vi "SavePosition_KCubeDCServo.vi"(4 "start/stop write":bool, 5 "init file":bool, 7 "Device":refnum<k24>, 8 "state in":T1(ring), 9 "filename save":string="D:\\Victor Sun\\optical trap control\\output_test\\testposition", 10 "folder path save":path, 11 "Byte Stream File in":refnum<file>) -> (0 "state out":T1(ring), 2 "current state":string, 3 "Byte Stream File out":refnum<file>)   [LabVIEW 2019]
doc: "saves datetime, position value, and isdevicebusy for dcservo motor"
uses:
  D:/Victor Sun/optical trap control/Kinesis/ThorLabs.MotionControl.KCube.DCServoCLI.dll
  Kinesis/ThorLabs.MotionControl.KCube.DCServoCLI.dll
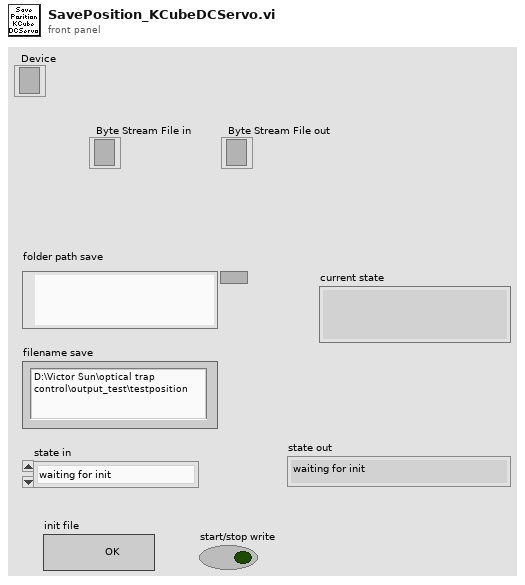
[diagram p1: front panel]
types:
  T1 = enum16{"waiting for init", "init", "waiting for write", "write", "stop", ""}
  T2 = enum16{"open", "replace", "create", "open or create", "replace or create", "replace or create with confirmation"}
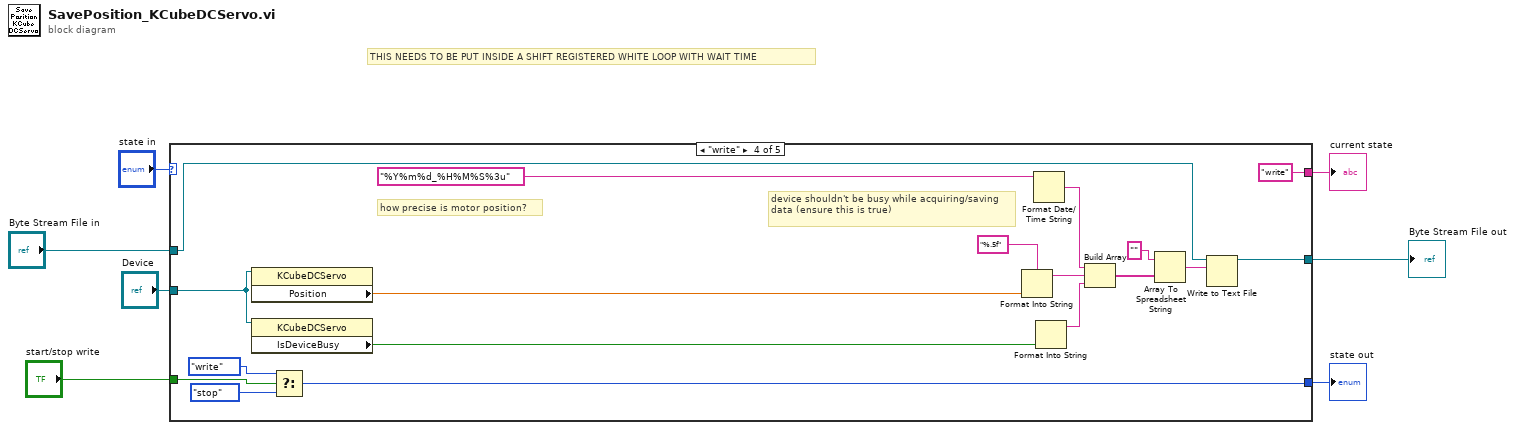
[diagram p0: block diagram]
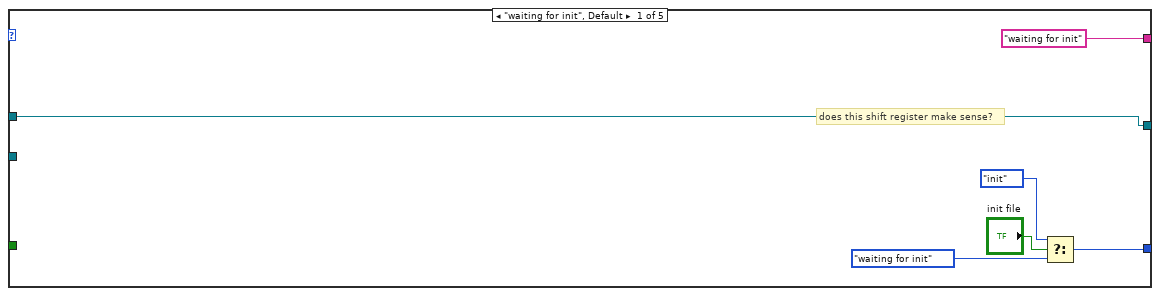
[diagram p2: hidden frame]
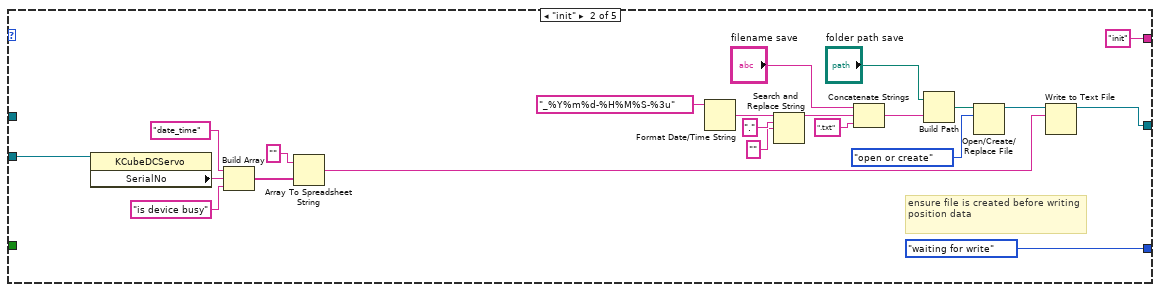
[diagram p3: hidden frame]
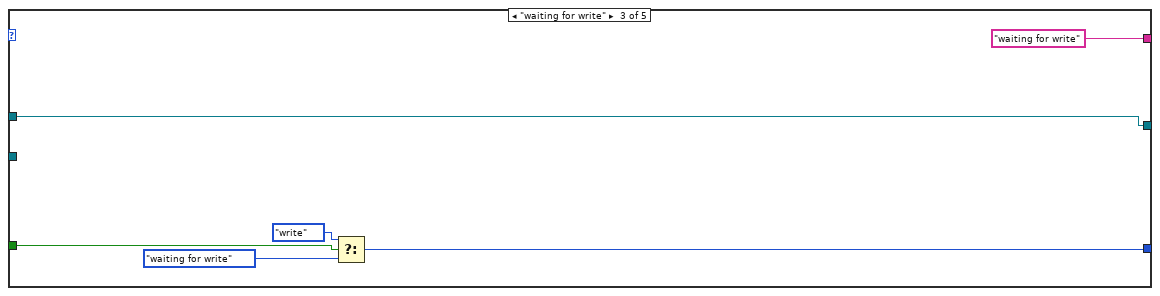
[diagram p4: hidden frame]
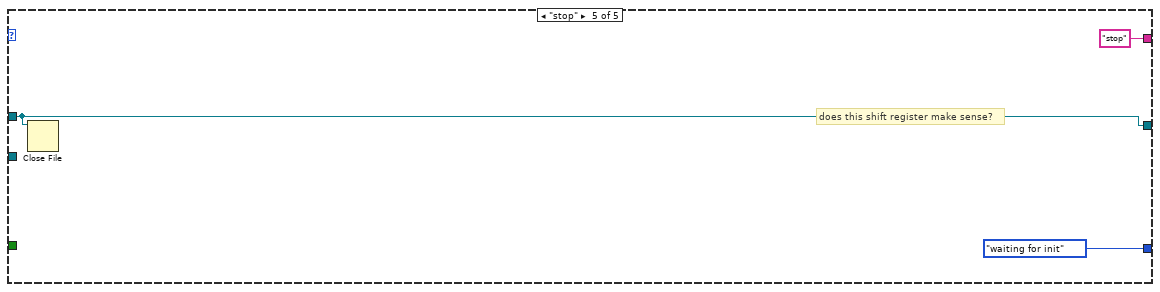
[diagram p5: hidden frame]
diagram:
  # "THIS NEEDS TO BE PUT INSIDE A SHIFT REGISTERED WHITE LOOP WITH WAIT TIME"
  n1 = case shown="\"write\"" "state in" {
    tunnel: [w12 T1."waiting for write" w40 w58 T1."waiting for init"] -> w2
    tunnel: ["waiting for init" ("String") "init" ("String") "waiting for write" ("String") "write" ("String") "stop" ("String")] -> w3
    tunnel: "Device" -> [_ w17 _ w56 _]
    tunnel: [w8 w16 w37 w55 w60] -> w5
    tunnel: "Byte Stream File in" -> [w8 _ w37 w57 w60]
    tunnel: "start/stop write" -> [_ _ w36 w44 _]
    frame "waiting for init", Default {
      # "does this shift register make sense?"
      n2 = Select(t=T1."init", s="init file", f=T1."waiting for init") -> (s? t:f=w12:T1)
    }
    frame "init" {
      # "ensure file is created before writing position data"
      n3 = property class="KCubeDCServo"(reference=w17) -> ("SerialNo"=w19:string)  [unwired: 1 in, 2 out]
      n4 = Build Array("date_time", w19, "is device busy" ("element")) -> (w18:string[])
      n5 = Array To Spreadsheet String(array=w18, 3:"" ("format string")) -> (spreadsheet string=w32:string)  [unwired: 1 in]
      n6 = Format Date/Time String(time format string (%c)="_%Y%m%d-%H%M%S-%3u") -> (date/time string=w27:string)  [unwired: 2 in]
      n7 = Search and Replace String(input string=w27, search string=".", replace string="" ("replace string (\"\")")) -> (result string=w28:string)  [unwired: 5 in, 3 out]
      n8 = Concatenate Strings("filename save", w28, ".txt" ("result string")) -> (w30:string)
      n9 = Build Path(base path="folder path save", name or relative path=w30) -> (appended path=w31:path)
      n10 = Open/Create/Replace File(file path (use dialog)=w31, operation (0:open)=T2."open or create") -> (refnum out=w33:refnum<file>)  [unwired: 4 in, 2 out]
      n11 = Write to Text File(file (use dialog)=w33, text=w32) -> (refnum out=w16:refnum<file>)  [unwired: 2 in, 2 out]
    }
    frame "waiting for write" {
      n12 = Select(t=T1."write", s=w36, f=T1."waiting for write") -> (s? t:f=w40:T1)
    }
    frame "write" {
      # "device shouldn't be busy while acquiring/saving data (ensure this is true)"
      # "how precise is motor position?"
      n13 = property class="KCubeDCServo"(reference=w56) -> ("Position"=w53:dbl)  [unwired: 1 in, 2 out]
      n14 = property class="KCubeDCServo"(reference=w56) -> ("IsDeviceBusy"=w46:bool)  [unwired: 1 in, 2 out]
      n15 = Select(t=T1."write", s=w44, f=T1."stop") -> (s? t:f=w58:T1)
      n16 = Format Into String(format string="%.5f", w53) -> (resulting string=w50:string)  [unwired: 2 in, 1 out]
      n17 = Format Date/Time String(time format string (%c)="%Y%m%d_%H%M%S%3u") -> (date/time string=w51:string)  [unwired: 2 in]
      n18 = Format Into String(w46) -> (resulting string=w45:string)  [unwired: 3 in, 1 out]
      n19 = Build Array(w51, w50, w45) -> (w49:string[])
      n20 = Array To Spreadsheet String(array=w49, 3:"" ("format string")) -> (spreadsheet string=w48:string)  [unwired: 1 in]
      n21 = Write to Text File(file (use dialog)=w57, text=w48) -> (refnum out=w55:refnum<file>)  [unwired: 2 in, 2 out]
    }
    frame "stop" {
      # "does this shift register make sense?"
      n22 = Close File(refnum=w60) -> ()  [unwired: 1 in, 2 out]
    }
  }
  "Byte Stream File out" <- w5
  "current state" <- w3
  "state out" <- w2
